vi "al_dmm_read.vi"(0 "DMM TSM In":T1, 11 "error in":errorcluster) -> (4 "measurement":dbl[](array[numeric]), 15 "error out":errorcluster)   [LabVIEW 2019]
uses:
  Instrument Control/DMM/Pin Map/TSM DMM.ctl
  <vilib>/NI_TestStand_SemiconductorModule/NI_TestStand_Semiconductor_Module.lvlibp/PinMap/PinQueryContext/MultiplePinMultipleSessionQueryContext/MultiplePinMultipleSessionQueryContext.lvclass
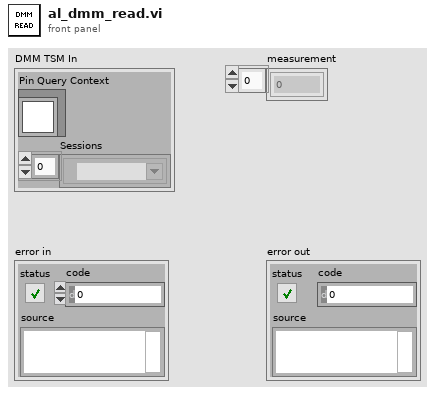
[diagram p1: front panel]
types:
  T1 = typedef "TSM DMM.ctl" = cluster{"Pin Query Context":refnum<class "MultiplePinMultipleSessionQueryContext.lvclass">, "Sessions":refnum<k15>[]}
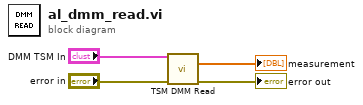
[diagram p0: block diagram]
diagram:
  n1 = call "TSM DMM Read.vi"("DMM TSM In"="DMM TSM In", "error in"="error in") -> ("measurement"=→"measurement":dbl[], "error out"=→"error out":errorcluster)  [unwired: 11 in, 1 out]
